vi "Config Trig Mode and Source.vi"(0 "VISA resource name":refnum<visa-resource-name>, 5 "Trigger Mode(0: OFF)":u16(ring) items=["OFF", "AUTO", "AT-LEVEL", "NORMAL", "HF AUTO", "HF NORMAL"], 7 "Source(1: CH1)":u16(ring)=1 items=["Ext", "CH1", "CH2", "CH3", "CH4", "CH5", "CH6", "CH7", "CH8"], 11 "error in (no error)":errorcluster) -> (4 "VISA resource name out":refnum<visa-resource-name>, 15 "error out":errorcluster)   [LabVIEW 2013, in "Yokogawa.lvlib" / "Yokogawa PZ4000.lvlib"]
doc: "This VI sends the Simple Trigger and Trigger Mode Control command to the PZ4000.\nConfiguration Functions are Trigger Mode, Source."
uses:
  Yokogawa PZ4000.lvlib
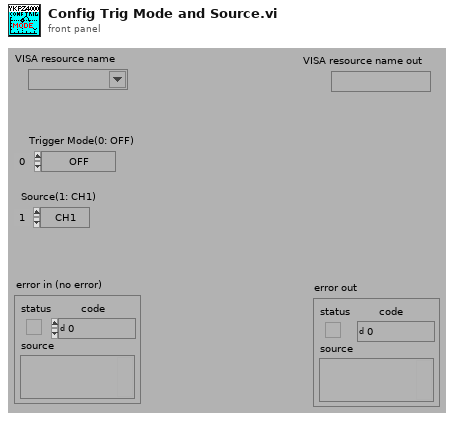
[diagram p1: front panel]
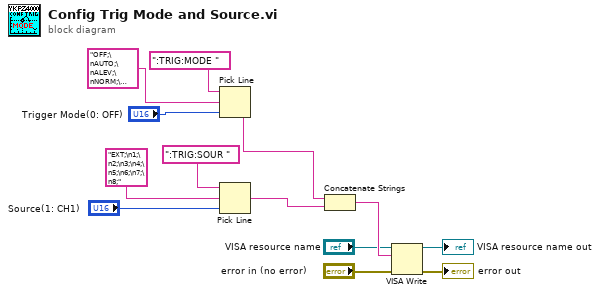
[diagram p0: block diagram]
diagram:
  n1 = Pick Line(string ("")=":TRIG:MODE ", multi-line string="OFF;\nAUTO;\nALEV;\nNORM;\nHFA;\nHFN;", line index="Trigger Mode(0: OFF)") -> (output string=w2:string)
  n2 = Pick Line(string ("")=":TRIG:SOUR ", multi-line string="EXT;\n1;\n2;\n3;\n4;\n5;\n6;\n7;\n8;", line index="Source(1: CH1)") -> (output string=w1:string)
  n3 = Concatenate Strings(w2, w1) -> (w10:string)
  n4 = VISA Write(VISA resource name="VISA resource name", write buffer=w10, error in (no error)="error in (no error)") -> (VISA resource name out=→"VISA resource name out":refnum<visa-resource-name>, error out=→"error out":errorcluster)  [unwired: 1 out]
